vi "Remove_EQE_and_Indep_if_manual.vi"(11 "Measurement queue in":T1(array[cluster]) {"Pixel to measure" items=["All", "1", "2", "3", "4", "5", "6", "7", "8"]}) -> (3 "Measurement queue out":T1(array[cluster]) {"Pixel to measure" items=["All", "1", "2", "3", "4", "5", "6", "7", "8"]})   [LabVIEW 2011]
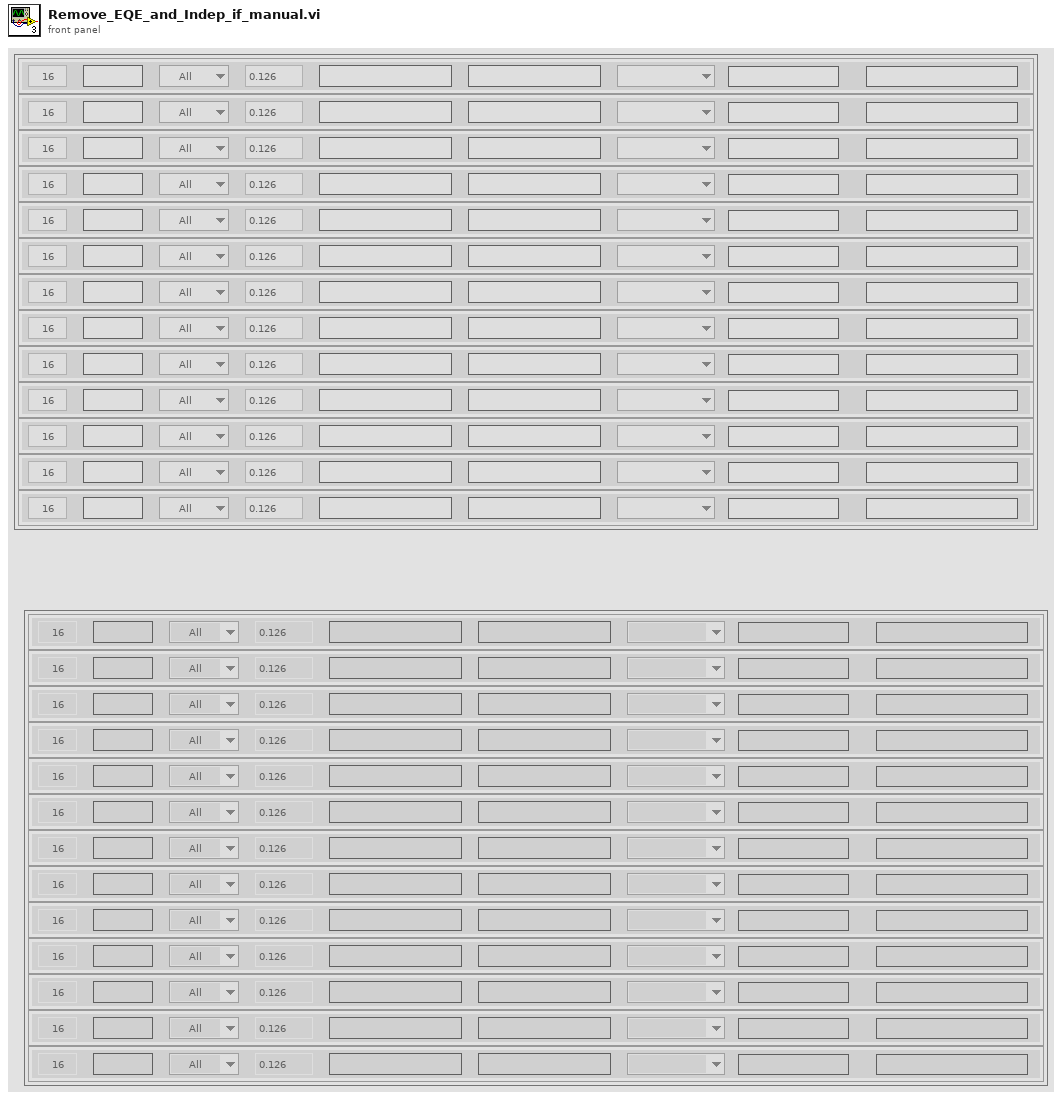
[diagram p1: front panel]
types:
  T1 = cluster{"Cell Position":i32, "Cell Label":string, "Pixel to measure":u16, "Area (cm^2)":dbl, "Variable":string, "Variable value":string, "Scan settings in queue":u16, "Light or dark":string, "Measurement type":string}[]
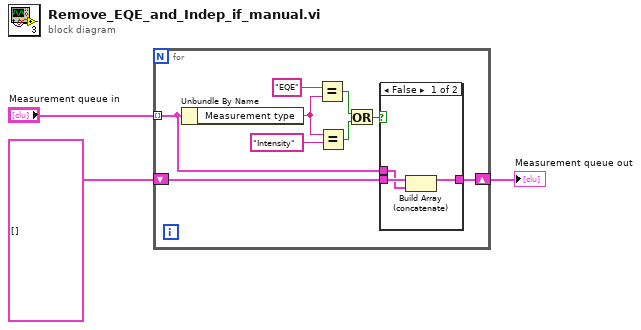
[diagram p0: block diagram]
diagram:
  n1 = for {
    tunnel: "Measurement queue in" -> [w4] mode=indexing
    shift-right: [w6] -> w2
    shift-left: T1 [] ("Measurement queue out") -> [w5]
    n2 = Unbundle By Name(w4) -> ("Measurement type"=w10:string)
    n3 = Equal?(x="EQE" ("element"), y=w10) -> (x = y?=w9:bool)
    n4 = Equal?(x=w10, y="Intensity" ("element")) -> (x = y?=w8:bool)
    n5 = Or(x=w9, y=w8) -> (x .or. y?=w7:bool)
    n6 = case shown="False" w7 {
      tunnel: [w15 w16] -> w6
      tunnel: w5 -> [w14 w16]
      tunnel: w4 -> [w13 _]
      frame False {
        n7 = Build Array (concatenate)(w14, w13) -> (w15:T1)
      }
      frame True {
      }
    }
  }
  "Measurement queue out" <- w2
